vi "activeCameras.vi"(7 "action":T5, 8 "error in (no error)":errorcluster, 11 "cameras":T1[](array[typedef])) -> (0 "error out":errorcluster, 3 "cameras":T1[](array[typedef]))   [LabVIEW 2017, in "VisionWebServiceData.lvlib"]
uses:
  VisionWebServiceData.lvlib
  action.ctl
  <vilib>/addons/InsightCM/Devices/Shared/Ir/IrAcquisition/controls/camera.ctl
  <vilib>/userdefined/High Color/IMAQdx.ctl
  <vilib>/vision/Image Controls.llb/IMAQ Image.ctl
  <vilib>/addons/PointValueMap/controls/PointMap.ctl
  <vilib>/addons/InsightCM/Devices/Shared/Ir/IrAcquisition/IrAcquisition.lvlib
  <vilib>/addons/PointValueMap/PointValueMap.lvlib
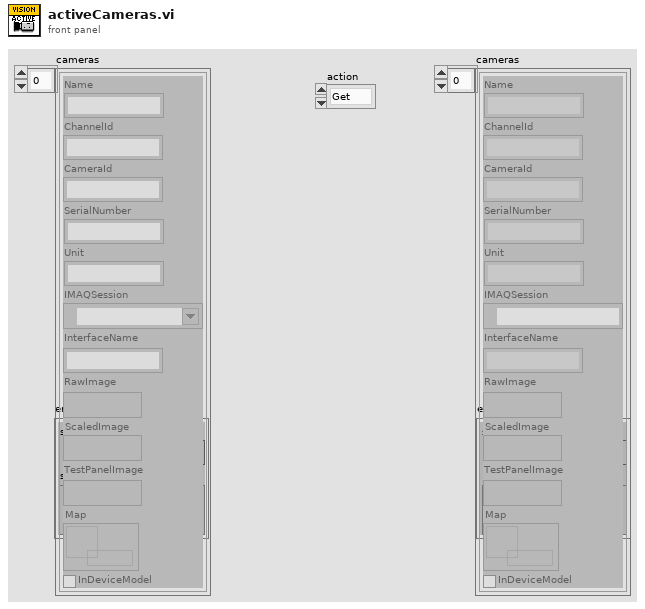
[diagram p1: front panel]
types:
  T1 = typedef "IrAcquisition.lvlib/camera.ctl" = cluster{"Name":string, "ChannelId":string, "CameraId":string, "SerialNumber":string, "Unit":string, "IMAQSession":T2, "InterfaceName":string, "RawImage":T3, "ScaledImage":T3, "TestPanelImage":T3, "Map":T4, "InDeviceModel":bool}
  T2 = typedef "IMAQdx.ctl" = refnum<k21>
  T3 = typedef "IMAQ Image.ctl" = refnum<image>
  T4 = typedef "PointValueMap.lvlib/PointMap.ctl" = refnum<data-value>
  T5 = typedef "VisionWebServiceData.lvlib/action.ctl" = enum16{"Get", "Set"}
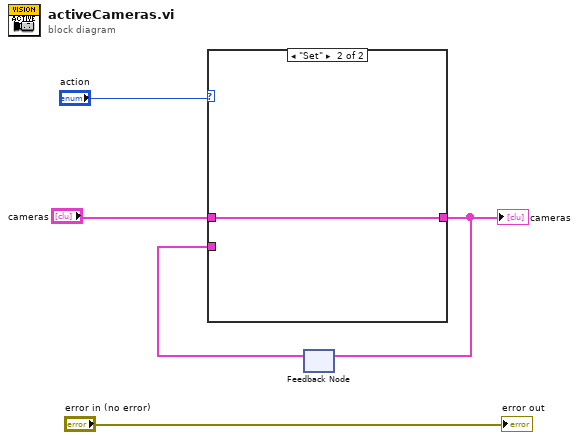
[diagram p0: block diagram]
diagram:
  n1 = feedback #1() -> (w3:T1[])  [unwired: 1 in]
  n2 = case shown="\"Set\"" "action" {
    tunnel: "cameras" -> [_ w7]
    tunnel: [w6 w7] -> w2
    tunnel: w3 -> [w6 _]
    frame "Get", Default {
    }
    frame "Set" {
    }
  }
  "cameras" <- w2
  n3 = feedback-in #1(w2) -> ()
  "error out" <- "error in (no error)"
